vi "show LIN Load Errors.vi"(4 "ABBRECHEN":T1 caption="CANCEL", 5 "loaded Setup Daten-Cluster":T3 caption="geladene Setup Daten", 6 "STARTEN":T1 caption="START", 7 "Ident Cluster":T2 caption="Ident", 11 "local Setup Daten-Cluster":T3 caption="lokale Setup Daten") -> (0 "CONTINUE":T1 caption="WEITER")   [LabVIEW 2020, in "Linearisierung v2.lvlib" / "SpanEinstellungen.lvlib"]
uses:
  SpanEinstellungen.lvlib
  LIN Loading Setup Data.ctl
  LIN Loading Errors.ctl
  Visualisierungs Elemente/Button.ctl
  Allgemein/allgemeine Sub-VIs.lvlib
panel:
  out "loaded Span different":string[][](array[string]) caption="geladener Spans anders"
  out "local Span different":string[][](array[string]) caption="lokaler Span anders"
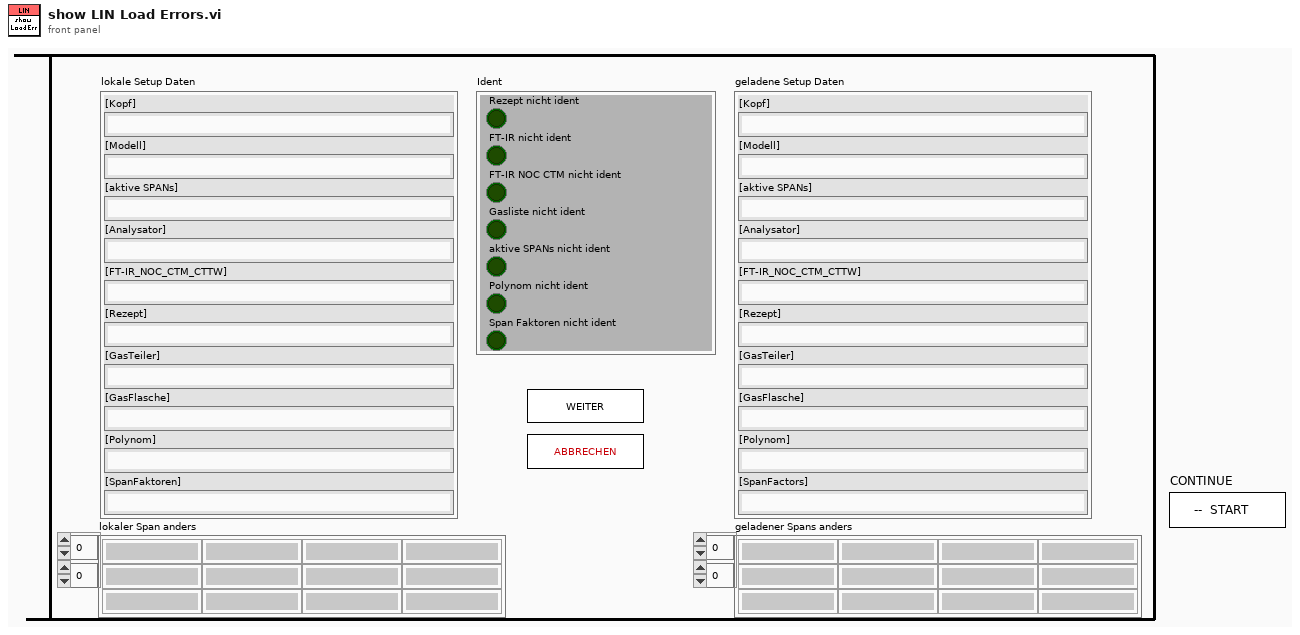
[diagram p1: front panel]
types:
  T1 = typedef "Button.ctl" = bool
  T2 = typedef "Linearisierung v2.lvlib/SpanEinstellungen.lvlib/LIN Loading Errors.ctl" = cluster{"Rezept nicht ident":bool, "FT-IR nicht ident":bool, "FT-IR NOC CTM nicht ident":bool, "Gasliste nicht ident":bool, "aktive SPANs nicht ident":bool, "Polynom nicht ident":bool, "Span Faktoren nicht ident":bool}
  T3 = typedef "Linearisierung v2.lvlib/SpanEinstellungen.lvlib/LIN Loading Setup Data.ctl" = cluster{"[Header]":string, "[Model]":string, "[active SPANs]":string, "[Analyser]":string, "[FT-IR_NOC_CTM_CTTW]":string, "[Recipie]":string, "[GasDivider]":string, "[GasBottle]":string, "[Polynomial]":string, "[SpanFactors]":string}
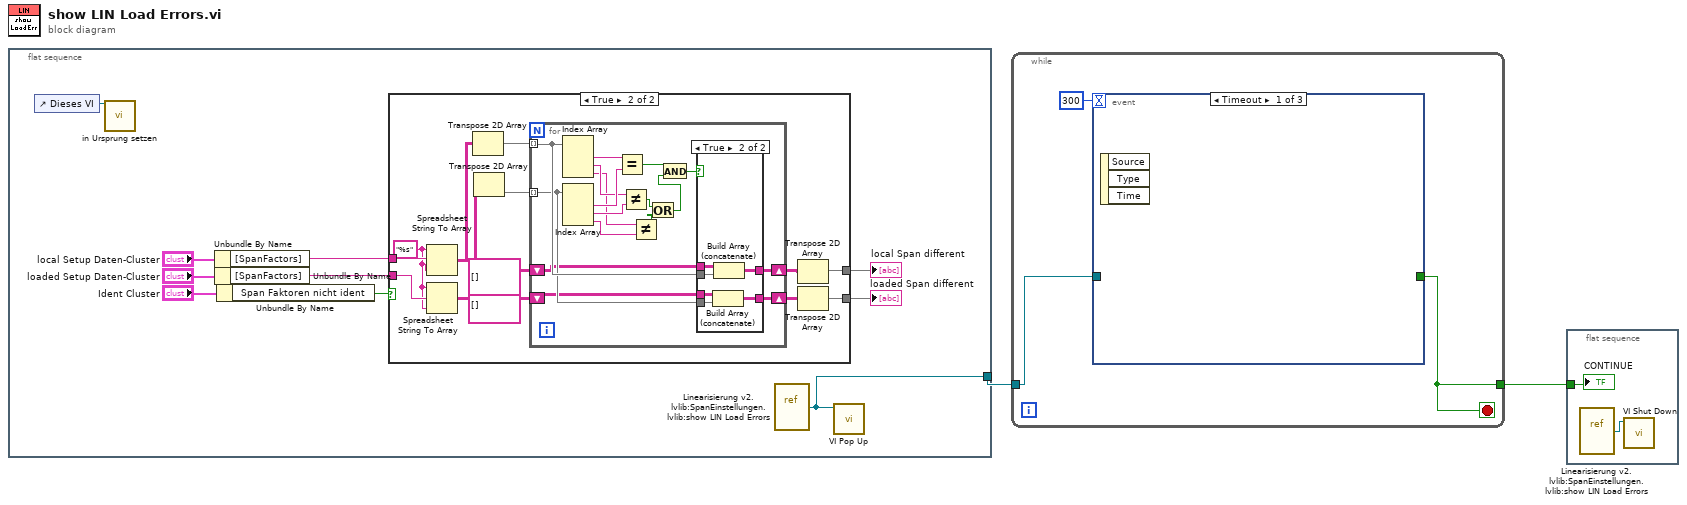
[diagram p0: block diagram]
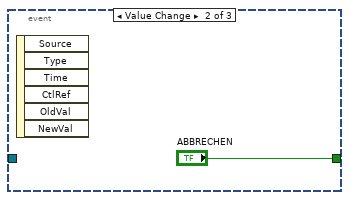
[diagram p4: hidden frame]
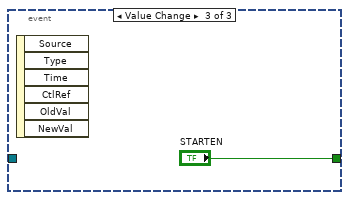
[diagram p5: hidden frame]
diagram:
  n1 = flat-sequence {
    tunnel: [w12] -> w1
    frame #0 {
      n2 = control-ref of="Dieses VI"() -> (w11:refnum<vi>)
      n3 = call "in Ursprung setzen.vi"("VI Referenz"=w11) -> ()  [unwired: 10 in, 1 out]
      n4 = Unbundle By Name("local Setup Daten-Cluster") -> ("[SpanFactors]"=w6:string)
      n5 = Unbundle By Name("loaded Setup Daten-Cluster") -> ("[SpanFactors]"=w5:string)
      n6 = Unbundle By Name("Ident Cluster") -> ("Span Faktoren nicht ident"=w9:bool)
      n7 = case shown="True" w9 {
        tunnel: w6 -> [_ w25]
        tunnel: w5 -> [_ w24]
        tunnel: [_ w15] -> w4
        tunnel: [_ w13] -> w3
        frame False {
        }
        frame True {
          w23 = "%s" ("Format-String")
          n8 = Spreadsheet String To Array(format string=w23, spreadsheet string=w25, array type (2D Dbl)=w23) -> (array=w22:string[][])  [unwired: 1 in]
          n9 = Spreadsheet String To Array(format string=w23, spreadsheet string=w24, array type (2D Dbl)=w23) -> (array=w21:string[][])  [unwired: 1 in]
          n10 = Transpose 2D Array(2D array=w22) -> (transposed array=w20:string[][])
          n11 = Transpose 2D Array(2D array=w21) -> (transposed array=w19:string[][])
          n12 = for {
            tunnel: w20 -> [w34] mode=indexing
            tunnel: w19 -> [w32] mode=indexing
            shift-right: [w33] -> w16
            shift-left: string[][] [] -> [w30]
            shift-right: [w31] -> w14
            shift-left: string[][] [] -> [w29]
            n13 = Index Array(array=w34) -> (element #1=w42:string, element #2=w40:string, element #3=w38:string)  [unwired: 3 in]
            n14 = Index Array(array=w32) -> (element #1=w41:string, element #2=w39:string, element #3=w37:string)  [unwired: 3 in]
            n15 = Equal?(x=w42, y=w41) -> (x = y?=w36:bool)
            n16 = Not Equal?(x=w40, y=w39) -> (x != y?=w28:bool)
            n17 = Not Equal?(x=w38, y=w37) -> (x != y?=w27:bool)
            n18 = Or(x=w28, y=w27) -> (x .or. y?=w26:bool)
            n19 = And(x=w36, y=w26) -> (x .and. y?=w35:bool)
            n20 = case shown="True" w35 {
              tunnel: w34 -> [_ w50]
              tunnel: [w44 w49] -> w33
              tunnel: w32 -> [_ w48]
              tunnel: [w43 w47] -> w31
              tunnel: w30 -> [w44 w46]
              tunnel: w29 -> [w43 w45]
              frame False {
              }
              frame True {
                n21 = Build Array (concatenate)(w45, w48) -> (w47:string[][])
                n22 = Build Array (concatenate)(w46, w50) -> (w49:string[][])
              }
            }
          }
          n23 = Transpose 2D Array(2D array=w16) -> (transposed array=w15:string[][])
          n24 = Transpose 2D Array(2D array=w14) -> (transposed array=w13:string[][])
        }
      }
      "local Span different" <- w4
      "loaded Span different" <- w3
      n25 = vi-ref "Linearisierung v2.lvlib:SpanEinstellungen.lvlib:show LIN Load Errors.vi"() -> (w12:refnum<vi>)
      n26 = call "VI Pop Up.vi"("VI Referenz"=w12) -> ()  [unwired: 10 in, 1 out]
    }
  }
  n27 = while {
    tunnel: [w52] -> w2
    tunnel: w1 -> [w51]
    stop <- w52 stop-if-true
    n28 = event shown="[0] Timeout" {
      selector: _ -> [_ _ _]
      dyn-events: _ -> [_ _ _]
      timeout: 300 -> [_ _ _]
      tunnel: [_ "ABBRECHEN" "STARTEN"] -> w52
      tunnel: w51 -> [_ _ _]
      event Timeout {
        n29 = event-data() -> ()  [unwired: 1 in, 3 out]
      }
      event Value Change {
        n30 = event-data() -> ()  [unwired: 1 in, 6 out]
      }
      event Value Change {
        n31 = event-data() -> ()  [unwired: 1 in, 6 out]
      }
    }
  }
  n32 = flat-sequence {
    tunnel: w2 -> [w56]
    frame #0 {
      n33 = vi-ref "Linearisierung v2.lvlib:SpanEinstellungen.lvlib:show LIN Load Errors.vi"() -> (w57:refnum<vi>)
      n34 = call "VI Shut Down.vi"("VI Referenz"=w57) -> ()  [unwired: 11 in]
      "CONTINUE" <- w56
    }
  }
